vi "EncoderDeadReckon.vi"(8 "Wheel Diameter":dbl, 9 "Diameter":dbl, 10 "Right Distance":dbl, 11 "Left Distance":dbl) -> (1 "Delta Theta":dbl, 2 "Delta Y":dbl, 3 "Delta X":dbl)   [LabVIEW 2013]
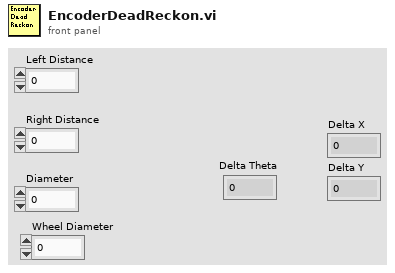
[diagram p1: front panel]
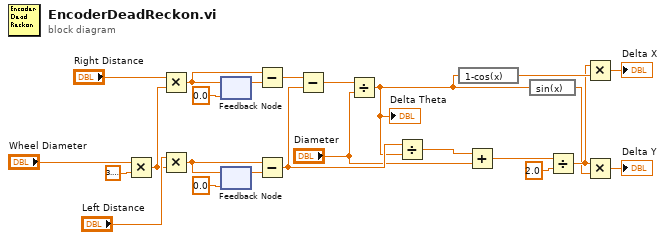
[diagram p0: block diagram]
diagram:
  n1 = Multiply(x="Wheel Diameter", y=3.141592653589793) -> (x*y=w20:dbl)
  n2 = Multiply(x="Right Distance", y=w20) -> (x*y=w15:dbl)
  n3 = Multiply(x="Left Distance", y=w20) -> (x*y=w14:dbl)
  n4 = feedback-in #1(w15) -> ()
  n5 = feedback #1(0.0) -> (w16:dbl)
  n6 = feedback-in #2(w14) -> ()
  n7 = feedback #2(0.0) -> (w17:dbl)
  n8 = Subtract(x=w15, y=w16) -> (x-y=w13:dbl)
  n9 = Subtract(x=w14, y=w17) -> (x-y=w11:dbl)
  n10 = Subtract(x=w13, y=w11) -> (x-y=w12:dbl)
  n11 = Divide(x=w12, y="Diameter") -> (x/y=w4:dbl)
  "Delta Theta" <- w4
  n12 = Divide(x=w11, y=w4) -> (x/y=w9:dbl)
  n13 = expression code="1-cos(x)"(w4) -> (w6:dbl)
  n14 = Add(x=w9, y="Diameter") -> (x+y=w8:dbl)
  n15 = expression code="sin(x)"(w4) -> (w2:dbl)
  n16 = Divide(x=w8, y=2.0) -> (x/y=w3:dbl)
  n17 = Multiply(x=w3, y=w6) -> (x*y=→"Delta X":dbl)
  n18 = Multiply(x=w3, y=w2) -> (x*y=→"Delta Y":dbl)
